vi "Funktionsgenerator - Kopie (2).vi"() -> ()   [LabVIEW 2017]
uses:
  <vilib>/Utility/error.llb/DialogType.ctl
  <vilib>/Analysis/3filter.llb/Filter Passband Type.ctl
  <vilib>/DAQmx/read.llb/DAQmx Read (Analog Wfm 1Chan NSamp).vi
  <vilib>/DAQmx/create/channels.llb/DAQmx Create Channel (AI-Voltage-Basic).vi
  <vilib>/DAQmx/configure/timing.llb/DAQmx Timing (Sample Clock).vi
  <vilib>/DAQmx/miscellaneous.llb/DAQmx Fill In Error Info.vi
  <vilib>/Analysis/3filter.llb/Chebyshev Filter (DBL).vi
  <vilib>/express/express analysis/Spectral/Block/exnSpectralBlock spectral measurements power poly.vi
  <vilib>/express/express analysis/Spectral/Block/exnSpectralBlock spectral measurements power WFM.vi
  <vilib>/Utility/file.llb/Write Delimited Spreadsheet (DBL).vi
  <vilib>/express/express analysis/Spectral/XNode/ExpressSpectralMeasurementsBlockNode.xnode
  <vilib>/Analysis/NI_AALBase.lvlib
panel:
  in  "Angenommene Trägerfrequenz":dbl
  in  "Speichern":bool
  out "Spektrum\nEingang":cluster{"f0":dbl, "df":dbl, "magnitude":dbl[]}(graph)
  out "Spektrum nach\nDemodulation":cluster{"f0":dbl, "df":dbl, "magnitude":dbl[]}(graph)
  out "Nach Demodulation":waveform(dbl)(graph)
  out "Eingang":waveform(dbl)(graph)
  in  "low cutoff freq: fl":dbl=10000.0 format="%0.4f"
  in  "Demodulator":T1(ring)
  out "Spektrum nach Tiefpass":cluster{"f0":dbl, "df":dbl, "magnitude":dbl[]}(graph)
  in  "stop":bool
  out "Nach Tiefpass":waveform(dbl)(graph)
  in  "minimum value":dbl=-10.0 format="%0.2f"
  in  "maximum value":dbl=10.0 format="%0.2f"
  in  "rate":dbl=40000.0 format="%0.2f"
  in  "physical channels":tag="Dev3/ai0"
  in  "samples per channel":i32=4000
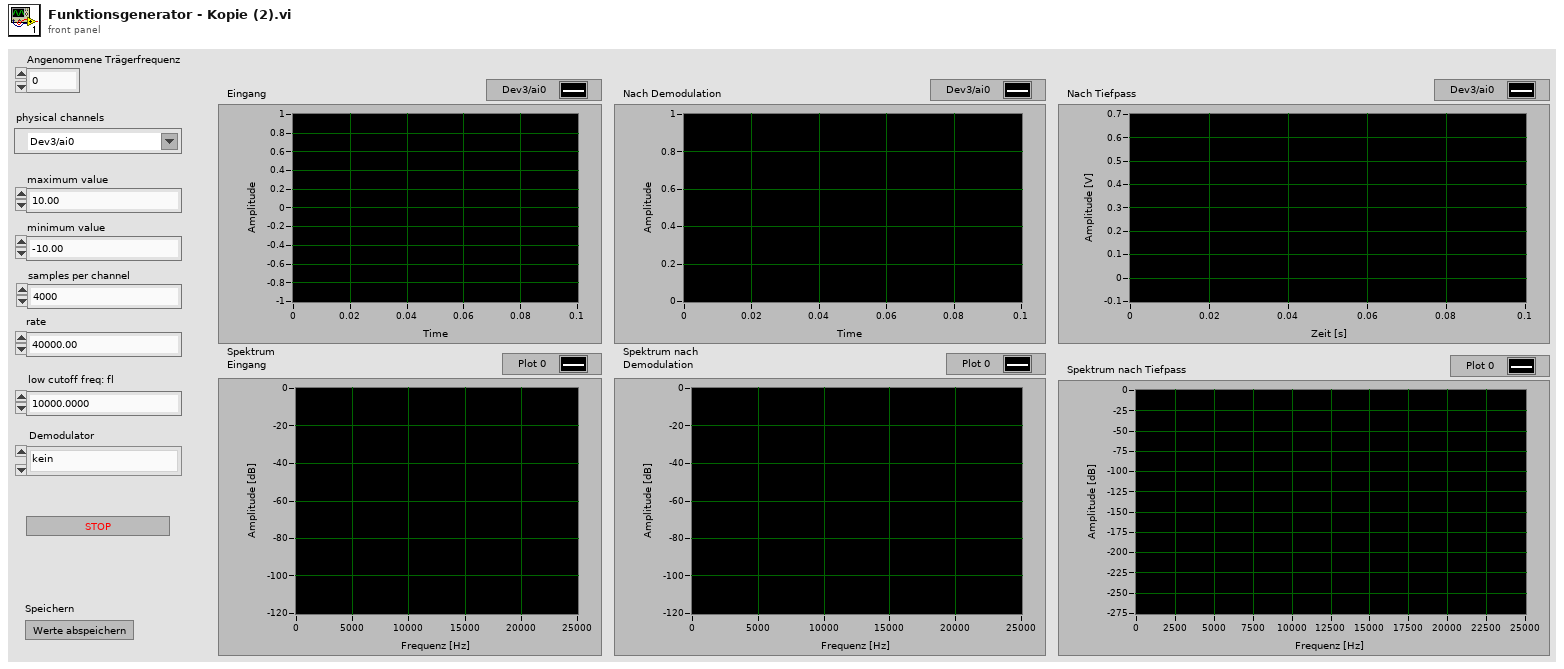
[diagram p1: front panel]
types:
  T1 = enum16{"kein", "Multiplikation mit Träger", "Quadrat", "Betrag"}
  T2 = typedef "NI_AALBase.lvlib/Filter Passband Type.ctl" = enum32{"Lowpass", "Highpass", "Bandpass", "Bandstop"}
  T3 = cluster{"averaging mode":u16, "weighting mode":u16, "number of averages":u32}
  T4 = cluster{"dB On (F)":bool, "unwrap phase (F)":bool, "convert to degree (F)":bool}
  T5 = typedef "DialogType.ctl" = u16
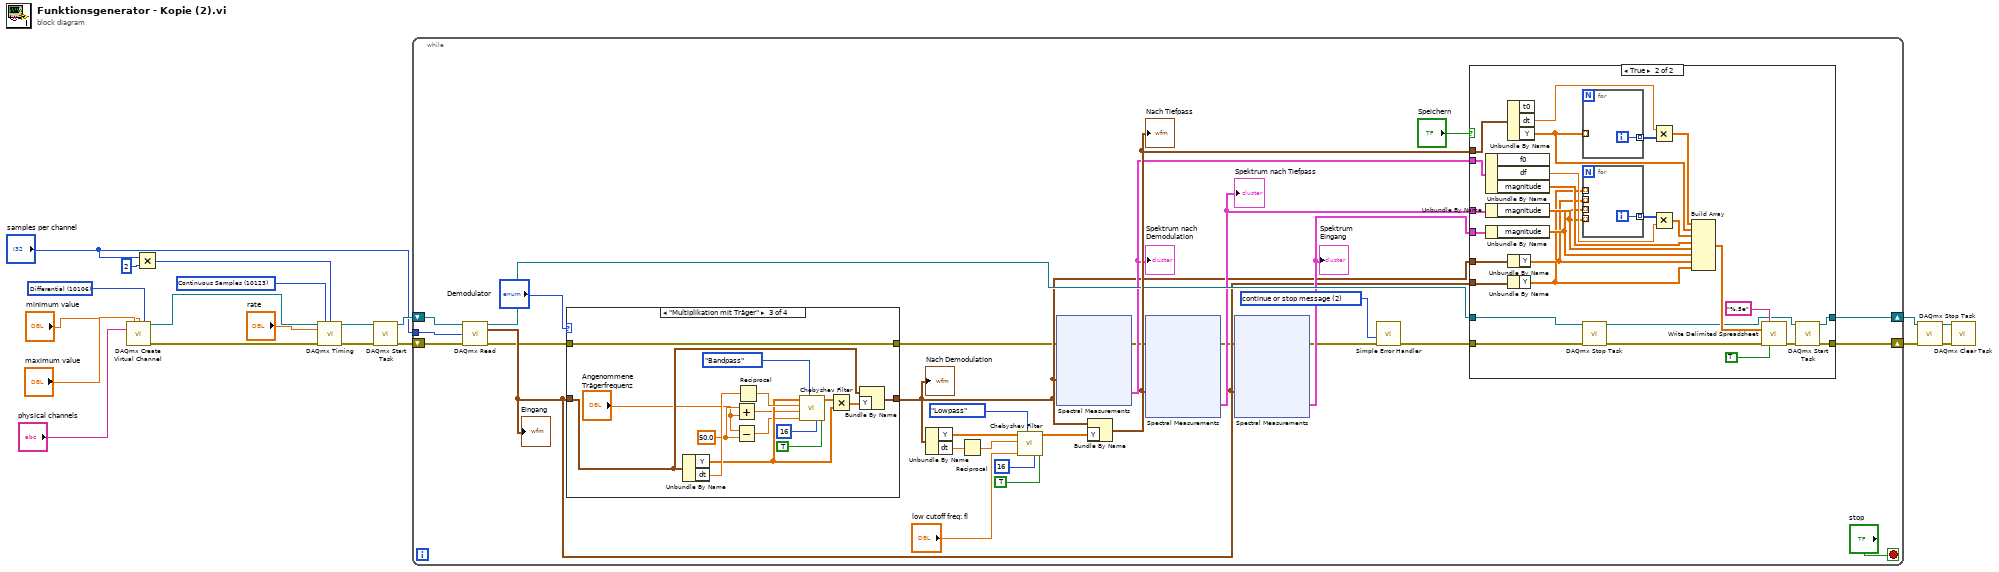
[diagram p0: block diagram]
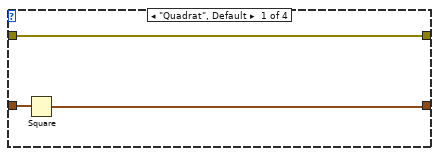
[diagram p3: hidden frame]
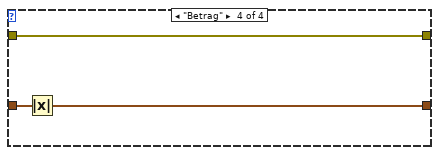
[diagram p5: hidden frame]
diagram:
  w5 = 10123 items=["Finite Samples"=10178, "Continuous Samples"=10123, "Hardware Timed Single Point"=12522] ("sample mode")
  w3 = 10106 items=["Default"=-1, "RSE"=10083, "NRSE"=10078, "Differential"=10106, "Pseudodifferential"=12529] ("input terminal configuration")
  n1 = call-poly <vilib>:"DAQmx Create Virtual Channel.vi"("maximum value"="maximum value", "minimum value"="minimum value", "input terminal configuration"=w3, "physical channels"="physical channels") -> ("task out"=w14:refnum<k21>, "error out"=w19:errorcluster)  [unwired: 10 in]
  n2 = Multiply(x="samples per channel", y=2 ("x*y")) -> (x*y=w2:i32)
  n3 = call-poly <vilib>:"DAQmx Timing.vi"("task/channels in"=w14, "sample mode"=w5, "samples per channel"=w2, "rate"="rate", "error in"=w19) -> ("task out"=w13:refnum<k21>, "error out"=w18:errorcluster)  [unwired: 9 in]
  n4 = call <vilib>:"DAQmx Start Task.vi"("task/channels in"=w13, "error in"=w18) -> ("task out"=w12:refnum<k21>, "error out"=w17:errorcluster)  [unwired: 12 in]
  n5 = while {
    shift-right: [w30] -> w16
    shift-left: w17 -> [w49]
    shift-right: [w31] -> w11
    shift-left: w12 -> [w48]
    tunnel: "samples per channel" -> [w46]
    stop <- "stop" stop-if-true
    w45 = T5 2 items=["no dialog", "OK message", "continue or stop message", "OK message + warnings", "continue/stop + warnings"] ("type of dialog (OK msg:1)")
    n6 = call-poly <vilib>:"DAQmx Read.vi"("task/channels in"=w48, "number of samples per channel"=w46, "error in"=w49) -> ("task out"=w32:refnum<k21>, "data"=w25:waveform(dbl), "error out"=w21:errorcluster)  [unwired: 10 in]
    "Eingang" <- w25
    n7 = case shown="\"Multiplikation mit Träger\"" "Demodulator" {
      tunnel: w25 -> [w102 w104 w109 w122]
      tunnel: [w101 w104 w114 w121] -> w26
      tunnel: w21 -> [w100 w103 w113 w120]
      tunnel: [w100 w103 w113 w120] -> w20
      frame "Quadrat", Default {
        n8 = Square(x=w102) -> (x^2=w101:waveform(dbl))
      }
      frame "kein" {
      }
      frame "Multiplikation mit Träger" {
        w107 = 50.0 ("x")
        n9 = Unbundle By Name(w109) -> ("Y"=w111:dbl[], "dt"=w115:dbl)
        n10 = Add(x=w107, y="Angenommene Trägerfrequenz") -> (x+y=w108:dbl)
        n11 = Subtract(x="Angenommene Trägerfrequenz", y=w107) -> (x-y=w105:dbl)
        n12 = Reciprocal(x=w115) -> (1/x=w117:dbl)
        n13 = call-poly <vilib>:"Chebyshev Filter.vi"("init/cont (init:F)"=TRUE, "order"=16, "filter type"=Filter_Passband_Type."Bandpass", "low cutoff freq: fl"=w105, "high cutoff freq: fh"=w108, "sampling freq: fs"=w117, "X"=w111) -> ("Filtered X"=w112:dbl[])  [unwired: 3 in, 1 out]
        n14 = Multiply(x=w112, y=w111) -> (x*y=w110:dbl[])
        n15 = Bundle By Name(cluster=w109, "Y"=w110) -> (w114:waveform(dbl))
      }
      frame "Betrag" {
        n16 = Absolute Value(x=w122) -> (abs(x)=w121:waveform(dbl))
      }
    }
    "Nach Demodulation" <- w26
    n17 = Unbundle By Name(w26) -> ("Y"=w41:dbl[], "dt"=w36:dbl)
    n18 = Reciprocal(x=w36) -> (1/x=w40:dbl)
    n19 = call-poly <vilib>:"Chebyshev Filter.vi"("init/cont (init:F)"=TRUE, "order"=16, "filter type"=Filter_Passband_Type."Lowpass", "low cutoff freq: fl"="low cutoff freq: fl", "sampling freq: fs"=w40, "X"=w41) -> ("Filtered X"=w37:dbl[])  [unwired: 4 in, 1 out]
    n20 = xnode "Spectral Measurements"("Signals"=w26, "error in (no error)"=w20) -> ("Power Spectrum"=w28:cluster{"f0":dbl, "df":dbl, "magnitude":dbl[]}, "error out"=w24:errorcluster)
    "Spektrum nach\nDemodulation" <- w28
    n21 = Bundle By Name(cluster=w26, "Y"=w37) -> (w34:waveform(dbl))
    "Nach Tiefpass" <- w34
    n22 = xnode "Spectral Measurements"("Signals"=w34, "error in (no error)"=w24) -> ("Power Spectrum"=w29:cluster{"f0":dbl, "df":dbl, "magnitude":dbl[]}, "error out"=w23:errorcluster)
    "Spektrum nach Tiefpass" <- w29
    n23 = xnode "Spectral Measurements"("Signals"=w25, "error in (no error)"=w23) -> ("Power Spectrum"=w27:cluster{"f0":dbl, "df":dbl, "magnitude":dbl[]}, "error out"=w22:errorcluster)
    "Spektrum\nEingang" <- w27
    n24 = call <vilib>:"Simple Error Handler.vi"("type of dialog (OK msg:1)"=w45, "error in (no error)"=w22) -> ("error out"=w33:errorcluster)  [unwired: 3 in, 4 out]
    n25 = case shown="True" "Speichern" {
      tunnel: w32 -> [w51 w68]
      tunnel: [w51 w62] -> w31
      tunnel: w33 -> [w50 w66]
      tunnel: [w50 w63] -> w30
      tunnel: w29 -> [_ w60]
      tunnel: w34 -> [_ w59]
      tunnel: w28 -> [_ w61]
      tunnel: w27 -> [_ w57]
      tunnel: w26 -> [_ w55]
      tunnel: w25 -> [_ w54]
      frame False {
      }
      frame True {
        n26 = Unbundle By Name(w61) -> ("df"=w73:dbl, "magnitude"=w77:dbl[])  [unwired: 1 out]
        n27 = Unbundle By Name(w60) -> ("magnitude"=w71:dbl[])
        n28 = Unbundle By Name(w57) -> ("magnitude"=w58:dbl[])
        n29 = Unbundle By Name(w59) -> ("dt"=w75:dbl, "Y"=w69:dbl[])  [unwired: 1 out]
        n30 = Unbundle By Name(w55) -> ("Y"=w53:dbl[])
        n31 = Unbundle By Name(w54) -> ("Y"=w52:dbl[])
        n32 = for {
          tunnel: [w81] -> w72 mode=indexing
          tunnel: w69 -> [_] mode=indexing
          i -> [w81]
        }
        n33 = for {
          tunnel: w71 -> [_] mode=indexing
          tunnel: [w80] -> w56 mode=indexing
          tunnel: w58 -> [_] mode=indexing
          tunnel: w53 -> [_] mode=indexing
          tunnel: w52 -> [_] mode=indexing
          i -> [w80]
        }
        n34 = call <vilib>:"DAQmx Stop Task.vi"("task/channels in"=w68, "error in"=w66) -> ("task out"=w67:refnum<k21>, "error out"=w65:errorcluster)  [unwired: 12 in]
        n35 = Multiply(x=w75, y=w72) -> (x*y=w74:dbl[])
        n36 = Multiply(x=w56, y=w73) -> (x*y=w70:dbl[])
        n37 = Build Array(w74, w69, w70, w77, w71, w58, w53, w52) -> (w76:dbl[][])
        n38 = call-poly <vilib>:"Write Delimited Spreadsheet.vi"("format (%.3f)"="%.5e", "2D data"=w76, "error in (no error)"=w65, "transpose? (no:F)"=TRUE) -> ("error out"=w64:errorcluster)  [unwired: 10 in, 1 out]
        n39 = call <vilib>:"DAQmx Start Task.vi"("task/channels in"=w67, "error in"=w64) -> ("task out"=w62:refnum<k21>, "error out"=w63:errorcluster)  [unwired: 12 in]
      }
    }
  }
  n40 = call <vilib>:"DAQmx Stop Task.vi"("task/channels in"=w11, "error in"=w16) -> ("task out"=w10:refnum<k21>, "error out"=w15:errorcluster)  [unwired: 12 in]
  n41 = call <vilib>:"DAQmx Clear Task.vi"("task in"=w10, "error in"=w15) -> ()  [unwired: 13 in, 1 out]
